vi "Get Channel Connection.vi"(8 "error in (no error)":errorcluster, 9 "Connection Type":string, 10 "Channel":string, 11 "Abstract Connection Lookup in":refnum<class "Abstract Connection Lookup.lvclass">) -> (0 "error out":errorcluster, 2 "Connected Channel":string, 3 "Abstract Connection Lookup out":refnum<class "Abstract Connection Lookup.lvclass">)   [LabVIEW 2020, in "Routing Templates.lvlib" / "Abstract Connection Lookup.lvclass"]
uses:
  Abstract Connection Lookup.lvclass
  Abstract Connection Lookup.lvclass/Abstract Connection Lookup.ctl
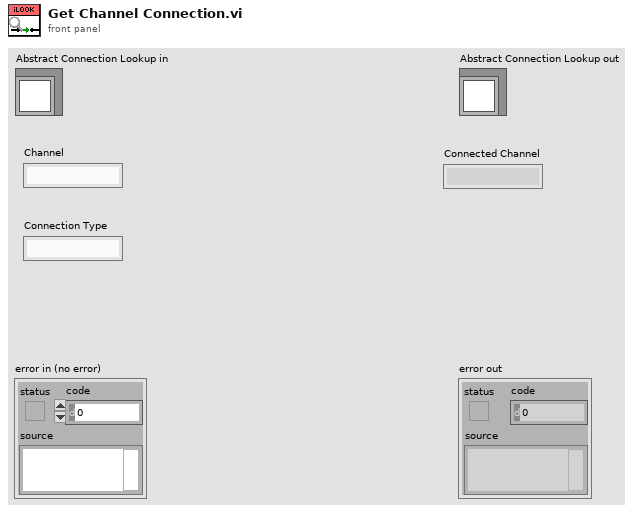
[diagram p1: front panel]
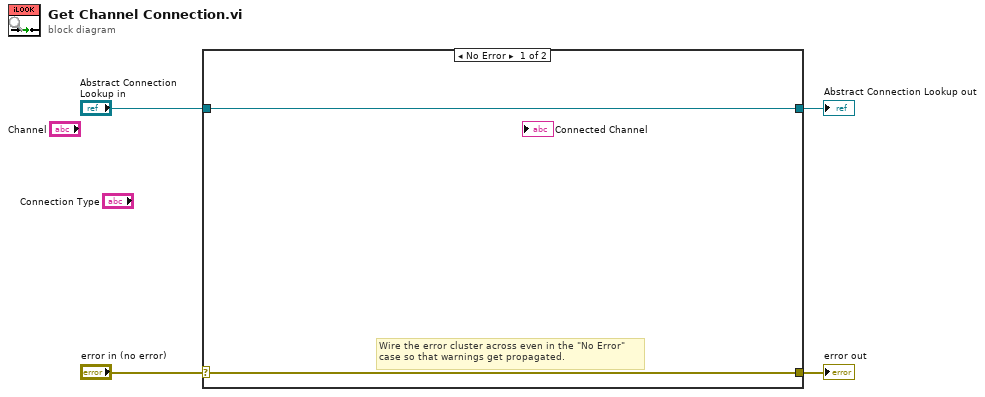
[diagram p0: block diagram]
diagram:
  n1 = case shown="No Error" "error in (no error)" {
    selector: "error in (no error)" -> [w5 w8]
    tunnel: [w5 w8] -> w3
    tunnel: [w6 w7] -> w1
    tunnel: "Abstract Connection Lookup in" -> [w6 w7]
    frame No Error {
      # "Wire the error cluster across even in the \"No Error\"\ncase so that warnings get propagated."
    }
    frame Error {
    }
  }
  "error out" <- w3
  "Abstract Connection Lookup out" <- w1
